vi "html actor loader.vi"(6 "Open Actor Core front panel? (T)":bool=TRUE, 8 "error in (no error)":errorcluster, 9 "Debug Alias":string, 10 "runtime (3000ms)":u32=3000, 11 "Actor":refnum<class "Actor.lvclass">) -> (0 "error out":errorcluster)   [LabVIEW 2021, in "AF Utils.lvlib"]
uses:
  AF Utils.lvlib
  System.Windows.Forms
  <vilib>/ActorFramework/Actor/Actor.lvclass
panel:
  in  "WebBrowser":refnum<k24>(container)
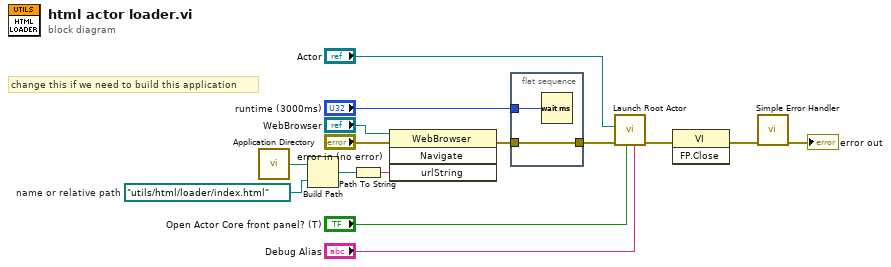
[diagram p0: block diagram]
diagram:
  w14 = path "utils/html/loader/index.html"  # name or relative path
  # "change this if we need to build this application"
  n1 = call <vilib>:"Application Directory.vi"() -> ("Application Directory"=w15:path)
  n2 = Build Path(base path=w15, name or relative path=w14) -> (appended path=w13:path)
  n3 = Path To String(path=w13) -> (string=w12:string)
  n4 = invoke class="WebBrowser" method="Navigate"(reference="WebBrowser", error in="error in (no error)", "urlString"=w12) -> (error out=w10:errorcluster)  [unwired: 1 in, 3 out]
  n5 = flat-sequence {
    tunnel: w10 -> [w17]
    tunnel: [w17] -> w9
    tunnel: "runtime (3000ms)" -> [w16]
    frame #0 {
      n6 = Wait (ms)(milliseconds to wait=w16) -> ()  [unwired: 1 out]
    }
  }
  n7 = call <vilib>:"Launch Root Actor.vi"("Debug Alias"="Debug Alias", "Open Actor Core front panel? (F)"="Open Actor Core front panel? (T)", "error in (no error)"=w9, "Actor"="Actor") -> ("error out"=w7:errorcluster)  [unwired: 6 in, 1 out]
  n8 = invoke class="VI" method="FP.Close"(error in=w7) -> (error out=w6:errorcluster)  [unwired: 2 in, 2 out]
  n9 = call <vilib>:"Simple Error Handler.vi"("error in (no error)"=w6) -> ("error out"=→"error out":errorcluster)  [unwired: 4 in, 4 out]
